vi "Read.vi"(8 "error in (no error)":errorcluster, 10 "Byte Count":u32, 11 "VISA resource name":refnum<visa-resource-name>) -> (0 "error out":errorcluster, 1 "Return Count":u32, 2 "Read Buffer":string, 3 "VISA resource name out":refnum<visa-resource-name>)   [LabVIEW 2013, in "LeCroy Wave Series.lvlib"]
doc: "Reads the specified number of bytes from the device or interface specified by VISA resource name and returns the data in read buffer. It is similar as VISA Read, but this is better for device communication over TCP/IP.\n\n<B>Note: </B>\n\nThis is a low-level Read VI that can be used to receive commands from the instrument for functionality not supported by the driver."
uses:
  LeCroy Wave Series.lvlib
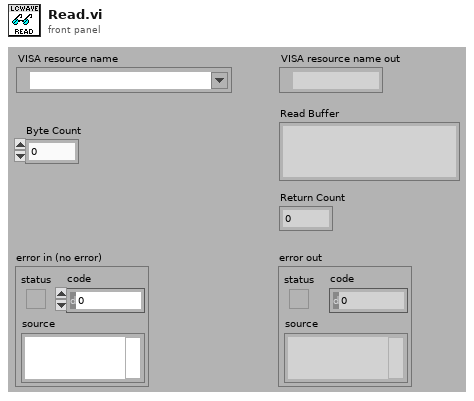
[diagram p1: front panel]
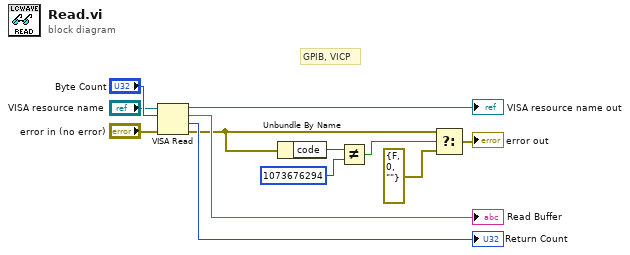
[diagram p0: block diagram]
diagram:
  # "GPIB, VICP"
  n1 = VISA Read(VISA resource name="VISA resource name", byte count="Byte Count", error in (no error)="error in (no error)") -> (VISA resource name out=→"VISA resource name out":refnum<visa-resource-name>, read buffer=→"Read Buffer":string, return count=→"Return Count":u32, error out=w3:errorcluster)
  n2 = Unbundle By Name(w3) -> ("code"=w7:i32)
  n3 = Not Equal?(x=w7, y=1073676294) -> (x != y?=w4:bool)
  n4 = Select(t=w3, s=w4, f=errorcluster {"status"=FALSE, "code"=0, "source"=""} ("error out")) -> (s? t:f=→"error out":errorcluster)
